vi "Check Enqueuer MAP.vi"(11 "Controller in":refnum<class "Controller.lvclass">) -> (3 "Enqueuer Map":variant)   [LabVIEW 2014, in "Controller.lvlib" / "Controller.lvclass"]
doc: "This VI checks the Enqueuer Map. If there are no enqueuers in the table, then the signal will be sent to the controller to shutdown. Otherwise, a copy of the Map is sent out."
uses:
  Controller.lvclass
  Controller.lvclass/Controller.ctl
  <vilib>/ActorFramework/Actor/Actor.lvclass/Actor.ctl
  <vilib>/ActorFramework/Message Enqueuer/Message Enqueuer.lvclass/Message Enqueuer.ctl
  <vilib>/ActorFramework/Message Enqueuer/Init from Existing Queue.vi
  <vilib>/ActorFramework/Message Enqueuer/Enqueue.vi
  <vilib>/ActorFramework/Message Priority Queue/Priority Enqueue.vi
  <vilib>/ActorFramework/Message Enqueuer/Message Enqueuer.lvclass
  <vilib>/ActorFramework/Stop Msg/Stop Msg.lvclass
  <vilib>/ActorFramework/Actor/Actor.lvclass
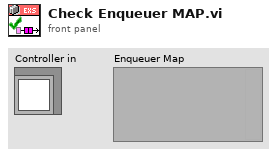
[diagram p1: front panel]
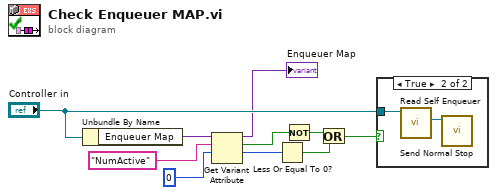
[diagram p0: block diagram]
diagram:
  n1 = Unbundle By Name("Controller in") -> ("Enqueuer Map"=w1:variant)
  n2 = Get Variant Attribute(Variant=w1, name="NumActive", default value (empty Variant)=i16 0) -> (duplicate Variant=→"Enqueuer Map":variant, found=w5:bool, value=w3:i16)  [unwired: 1 in, 1 out]
  n3 = Less Or Equal To 0?(x=w3) -> (x <= 0?=w4:bool)
  n4 = Not(x=w5) -> (.not. x?=w6:bool)
  n5 = Or(x=w6, y=w4) -> (x .or. y?=w7:bool)
  n6 = case shown="True" w7 {
    tunnel: "Controller in" -> [_ w11]
    frame False {
    }
    frame True {
      n7 = call <vilib>:"Read Self Enqueuer.vi"("Actor"=w11) -> ("Self Enqueuer"=w12:refnum<class "Message Enqueuer.lvclass">)  [unwired: 10 in]
      n8 = call <vilib>:"Send Normal Stop.vi"("Message Enqueuer"=w12) -> ()  [unwired: 10 in, 1 out]
    }
  }
